vi "O2 Leaktest FGV.vi"(6 "Aktion":T3, 8 "Textname:":string, 9 "Pfad:":path=path "D:/IAG_Data/Log", 10 "O2 Settings":T1 {"Grenzwert: Messgasdruck" format="%#.1f"; "Grenzwert: O2" format="%#.1f"; "Datenerfassungszeit:" format="%#.1f"; "Nullgas Aufschaltzeit:" format="%#.1f"; "Aufschaltpunkt" items=["Filterblock", "Analyzer directly", "PNS"]; "Kalibriergas" items=["Stickstoff", "CO", "C3H8", "CH4", "O2", "", "", "", "", "", "", "", ""]}) -> (0 "Textname:":string, 1 "Pfad:":path, 2 "O2 Settings":T1 {"Grenzwert: Messgasdruck" format="%#.1f"; "Grenzwert: O2" format="%#.1f"; "Datenerfassungszeit:" format="%#.1f"; "Nullgas Aufschaltzeit:" format="%#.1f"; "Aufschaltpunkt" items=["Filterblock", "Analyzer directly", "PNS"]; "Kalibriergas" items=["Stickstoff", "CO", "C3H8", "CH4", "O2", "", "", "", "", "", "", "", ""]})   [LabVIEW 2015]
uses:
  Allgemein/allgemeine Sub-VIs.lvlib
  Aktion FGV O2 Leak.ctl
  Visualisierungs Elemente/Auswahlfeld.ctl
  O2 Settings.ctl
  O2 Dichtheitstest.lvlib
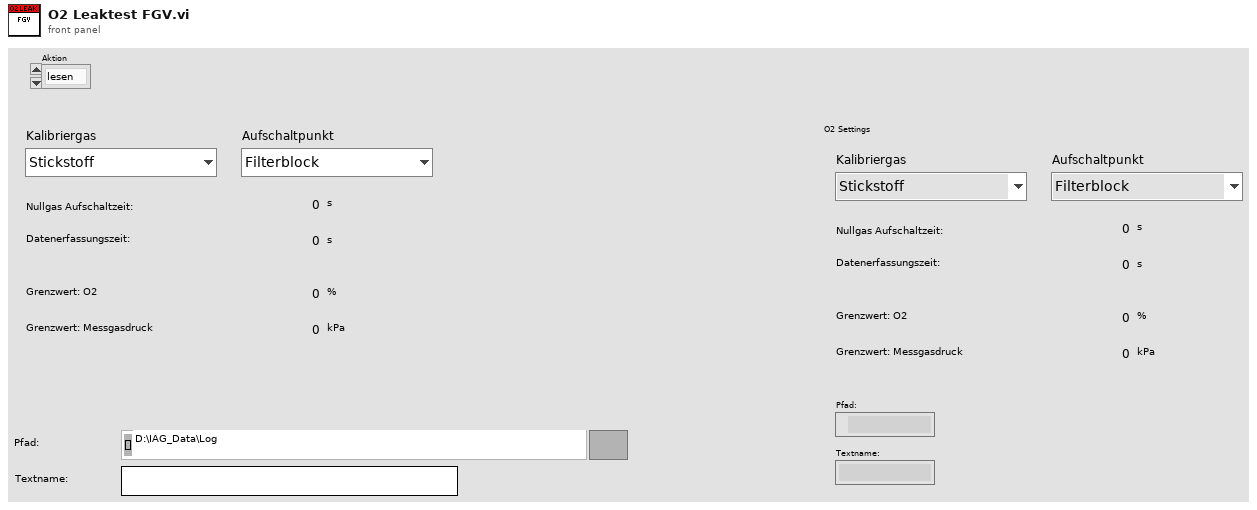
[diagram p1: front panel]
types:
  T1 = typedef "O2 Dichtheitstest.lvlib/O2 Settings.ctl" = cluster{"Kalibriergas":T2, "Aufschaltpunkt":T2, "Nullgas Aufschaltzeit:":sgl, "Datenerfassungszeit:":sgl, "Grenzwert: O2":sgl, "Grenzwert: Messgasdruck":sgl}
  T2 = typedef "Auswahlfeld.ctl" = u16
  T3 = typedef "Aktion FGV O2 Leak.ctl" = enum16{"lesen", "O2 settings", "Pfad", "Protokoll", "laden", "speichern"}
  T4 = cluster{"O2 Settings":T1, "Textname:":string, "Pfad:":path}
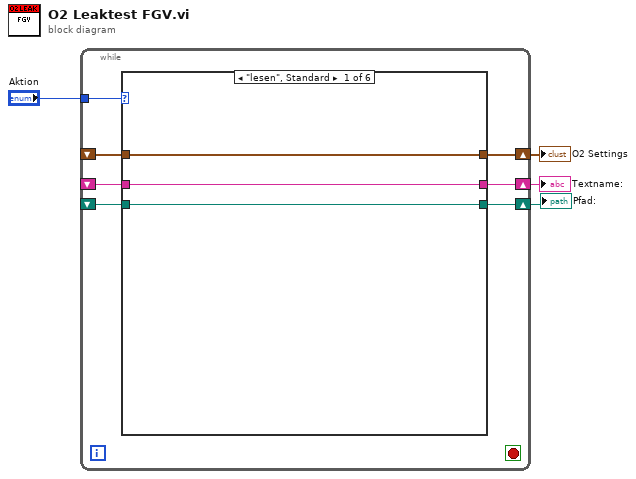
[diagram p0: block diagram]
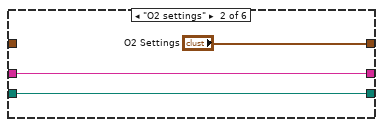
[diagram p2: hidden frame]
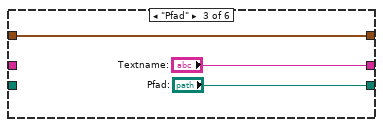
[diagram p3: hidden frame]
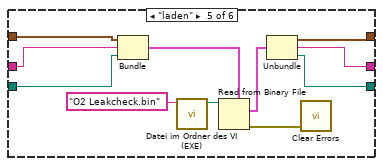
[diagram p5: hidden frame]
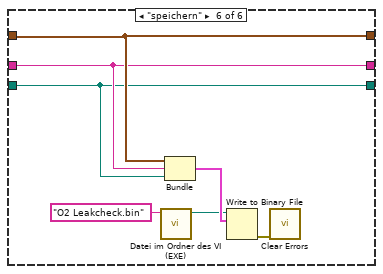
[diagram p6: hidden frame]
diagram:
  n1 = while {
    tunnel: "Aktion" -> [w11]
    shift-right: [w10] -> w3
    shift-left: _ -> [w9]
    shift-right: [w8] -> w2
    shift-left: _ -> [w7]
    shift-right: [w6] -> w1
    shift-left: _ -> [w5]
    stop <- _ stop-if-true
    n2 = case shown="\"lesen\", Standard" w11 {
      tunnel: [w14 "O2 Settings" w18 w23 w27 w37] -> w10
      tunnel: w9 -> [w14 _ w18 w23 w30 w37]
      tunnel: [w13 w16 "Textname:" w22 w26 w36] -> w8
      tunnel: w7 -> [w13 w16 _ w22 w29 w36]
      tunnel: [w12 w15 "Pfad:" w21 w25 w35] -> w6
      tunnel: w5 -> [w12 w15 _ w21 w28 w35]
      frame "lesen", Default {
      }
      frame "O2 settings" {
      }
      frame "Pfad" {
      }
      frame "Protokoll" {
      }
      frame "laden" {
        n3 = Bundle("O2 Settings"=w30, "Textname:"=w29, "Pfad:"=w28) -> (w33:T4)  [unwired: 1 in]
        n4 = call "Datei im Ordner des VI (EXE).vi"("Dateiname"="O2 Leakcheck.bin") -> ("Dateipfad im Ordner des Haupt-VIs"=w31:path)  [unwired: 8 in, 2 out]
        n5 = Read from Binary File(5:w33, 11:w31) -> (0:w24:errorcluster, 2:w34:T4)  [unwired: 4 in, 2 out]
        n6 = Unbundle(w34) -> ("O2 Settings"=w27:T1, "Textname:"=w26:string, "Pfad:"=w25:path)
        n7 = call <vilib>:"Clear Errors.vi"("error in (no error)"=w24) -> ()  [unwired: 5 in, 2 out]
      }
      frame "speichern" {
        n8 = call "Datei im Ordner des VI (EXE).vi"("Dateiname"="O2 Leakcheck.bin") -> ("Dateipfad im Ordner des Haupt-VIs"=w39:path)  [unwired: 8 in, 2 out]
        n9 = Bundle("O2 Settings"=w37, "Textname:"=w36, "Pfad:"=w35) -> (w41:T4)  [unwired: 1 in]
        n10 = Write to Binary File(file (use dialog)=w39, data=w41) -> (error out=w38:errorcluster)  [unwired: 4 in, 2 out]
        n11 = call <vilib>:"Clear Errors.vi"("error in (no error)"=w38) -> ()  [unwired: 5 in, 2 out]
      }
    }
  }
  "O2 Settings" <- w3
  "Textname:" <- w2
  "Pfad:" <- w1
